vi "Motor_AdjAoRange.vi"(8 "error in (no error)":errorcluster, 10 "FeedForwardVol":dbl[](array[numeric]), 11 "Motors_New in":refnum<class "MotorControl.lvclass">) -> (0 "error out":errorcluster, 2 "Adj AO Range":cluster{"output high":dbl, "output low":dbl}[](array[cluster]), 3 "Motors_New out":refnum<class "MotorControl.lvclass">)   [LabVIEW 2015, in "MotorControl.lvclass"]
uses:
  MotorControl.lvclass
  MotorControl.lvclass/MotorControl.ctl
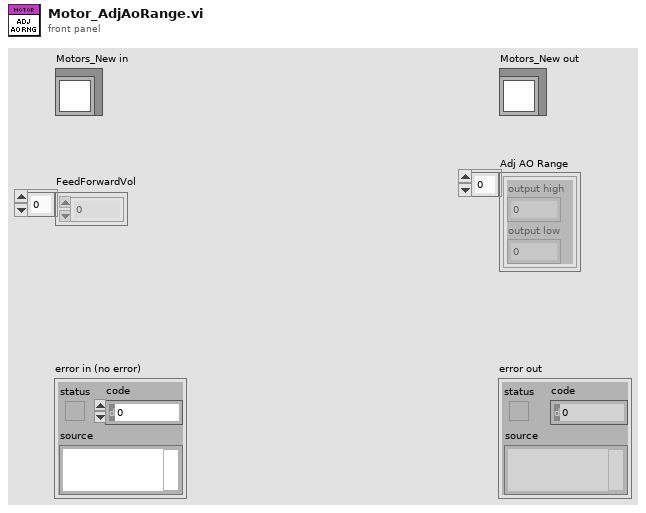
[diagram p1: front panel]
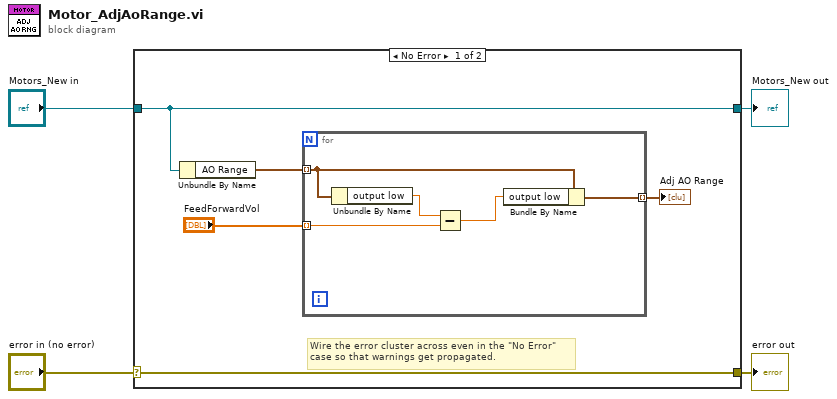
[diagram p0: block diagram]
diagram:
  n1 = case shown="No Error" "error in (no error)" {
    selector: "error in (no error)" -> [w9 w16]
    tunnel: [w9 w16] -> w3
    tunnel: [w8 w15] -> w1
    tunnel: "Motors_New in" -> [w8 w15]
    frame No Error {
      # "Wire the error cluster across even in the \"No Error\"\ncase so that warnings get propagated."
      n2 = Unbundle By Name(w8) -> ("AO Range"=w7:cluster{"output high":dbl, "output low":dbl}[])
      n3 = for {
        tunnel: w7 -> [w14] mode=indexing
        tunnel: "FeedForwardVol" -> [w12] mode=indexing
        tunnel: [w10] -> w5 mode=indexing
        n4 = Unbundle By Name(w14) -> ("output low"=w13:dbl)
        n5 = Subtract(x=w13, y=w12) -> (x-y=w11:dbl)
        n6 = Bundle By Name(cluster=w14, "output low"=w11) -> (w10:cluster{"output high":dbl, "output low":dbl})
      }
      "Adj AO Range" <- w5
    }
    frame Error {
    }
  }
  "error out" <- w3
  "Motors_New out" <- w1
